vi "GetSwitchOnlyPos.vi"(4 "error in (no error)":errorcluster, 7 "Circuit ID":i32=7201 format="%_4g") -> (0 "Error out":errorcluster, 3 "Position (0=open, 1=closed)":i32)   [LabVIEW 2012]
doc: "Reads a value from the 34980. \nGet switch position only, and not verify sense, paired, or pulse attributes"
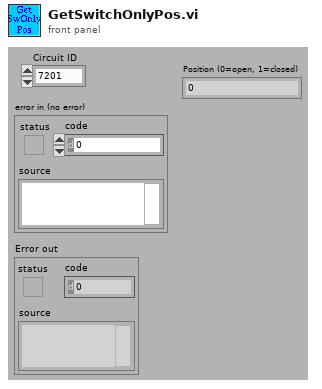
[diagram p1: front panel]
types:
  T1 = enum16{"N1911A", "Siggen", "34980a", "E4418B", "Rvp8"}
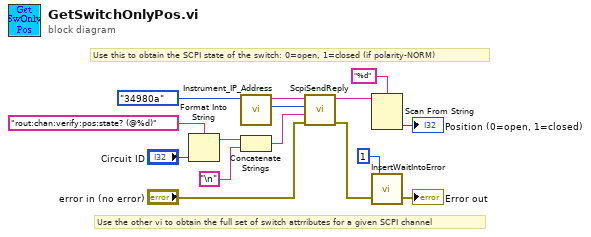
[diagram p0: block diagram]
diagram:
  # "Use the other vi to obtain the full set of switch attrributes for a given SCPI channel"
  # "Use this to obtain the SCPI state of the switch: 0=open, 1=closed (if polarity-NORM)"
  n1 = Format Into String(format string="rout:chan:verify:pos:state? (@%d)", "Circuit ID") -> (resulting string=w10:string)  [unwired: 2 in, 1 out]
  n2 = call "Instrument_IP_Address.vi"("Instrument"=T1."34980a") -> ("Port"=w1:u16, "IP Address"=w2:string)  [unwired: 9 in]
  n3 = Concatenate Strings(w10, "\n") -> (w8:string)
  n4 = call "ScpiSendReply.vi"("error in (no error)"="error in (no error)", "Command"=w8, "TCP port"=w1, "IP Address"=w2) -> ("Error out"=w7:errorcluster, "Reply"=w14:string)  [unwired: 5 in]
  n5 = Scan From String(format string="%d", input string=w14) -> (output 1=→"Position (0=open, 1=closed)":i32)  [unwired: 3 in, 3 out]
  n6 = call "InsertWaitIntoError.vi"("error in (no error)"=w7, "Wait (msecs)"=1) -> ("error out"=→"Error out":errorcluster)  [unwired: 1 in]
